vi "xijk_search_2D_table.vi"(8 "error in":errorcluster, 10 "sort array in":i32[](array[numeric]), 11 "all rows in":string[][](array[string])) -> (0 "error out":errorcluster, 3 "all rows out":string[][](array[string]))   [LabVIEW 2009, in "xijk_select_best_filter.lvlib"]
uses:
  xijk_select_best_filter.lvlib
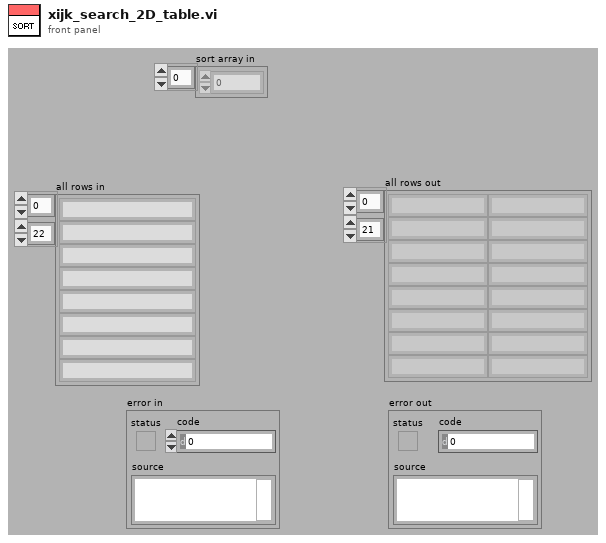
[diagram p1: front panel]
types:
  T1 = cluster{"all rows in[0]":string, "all rows in[1]":string, "all rows in[2]":string, "all rows in[3]":string, "all rows in[4]":string, "all rows in[5]":string, "all rows in[6]":string, "all rows in[7]":string, "all rows in[8]":string, "all rows in[9]":string, "all rows in[10]":string, "all rows in[11]":string, "all rows in[12]":string, "all rows in[13]":string, "all rows in[14]":string, "all rows in[15]":string, "all rows in[16]":string, "all rows in[17]":string, "all rows in[18]":string, "all rows in[19]":string, "all rows in[20]":string, "all rows in[21]":string, "all rows in[22]":string}
  T2 = cluster{"String":dbl, "all rows in":cluster{"all rows in[0]":string, "all rows in[1]":string, "all rows in[2]":string, "all rows in[3]":string, "all rows in[4]":string, "all rows in[5]":string, "all rows in[6]":string, "all rows in[7]":string, "all rows in[8]":string, "all rows in[9]":string, "all rows in[10]":string, "all rows in[11]":string, "all rows in[12]":string, "all rows in[13]":string, "all rows in[14]":string, "all rows in[15]":string, "all rows in[16]":string, "all rows in[17]":string, "all rows in[18]":string, "all rows in[19]":string, "all rows in[20]":string, "all rows in[21]":string, "all rows in[22]":string}}
  T3 = cluster{"String":dbl, "all rows in":cluster{"all rows in[0]":string, "all rows in[1]":string, "all rows in[2]":string, "all rows in[3]":string, "all rows in[4]":string, "all rows in[5]":string, "all rows in[6]":string, "all rows in[7]":string, "all rows in[8]":string, "all rows in[9]":string, "all rows in[10]":string, "all rows in[11]":string, "all rows in[12]":string, "all rows in[13]":string, "all rows in[14]":string, "all rows in[15]":string, "all rows in[16]":string, "all rows in[17]":string, "all rows in[18]":string, "all rows in[19]":string, "all rows in[20]":string, "all rows in[21]":string, "all rows in[22]":string}}[]
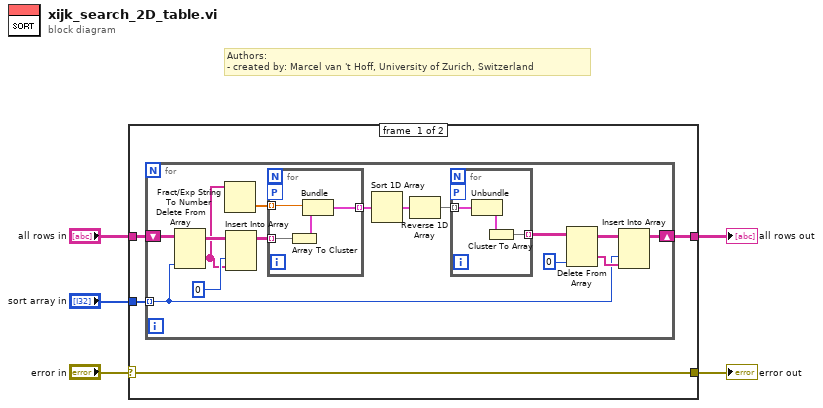
[diagram p0: block diagram]
diagram:
  # "Authors: \n- created by: Marcel van 't Hoff, University of Zurich, Switzerland"
  n1 = case shown="No Error" "error in" {
    selector: "error in" -> [w6 w32]
    tunnel: "sort array in" -> [w9 _]
    tunnel: "all rows in" -> [w8 _]
    tunnel: [w6 w32] -> w1
    tunnel: [w7 _] -> w2
    frame #0 {
      n2 = for {
        shift-right: [w16] -> w7
        shift-left: w8 -> [w13]
        tunnel: w9 -> [w14] mode=indexing
        n3 = Delete From Array(array=w13, index (col)=w14) -> (deleted portion=w12:string[], array with subset deleted=w22:string[][])  [unwired: 2 in]
        n4 = Fract/Exp String To Number(string=w12) -> (number=w11:dbl[])  [unwired: 3 in, 1 out]
        n5 = Insert Into Array(array=w22, index (col)=0 ("disabled index (col)"), new element=w12) -> (w17:string[][])  [unwired: 1 in]
        n6 = for {
          tunnel: w17 -> [w28] mode=indexing
          workers-P: _ -> [_]
          tunnel: w11 -> [w26] mode=indexing
          tunnel: [w25] -> w10 mode=indexing
          n7 = Array To Cluster(array=w28) -> (cluster=w27:T1)
          n8 = Bundle("String"=w26, "all rows in"=w27) -> (w25:T2)  [unwired: 1 in]
        }
        n9 = Sort 1D Array(array=w10) -> (sorted array=w23:T3)
        n10 = Reverse 1D Array(array=w23) -> (reversed array=w24:T3)
        n11 = for {
          tunnel: w24 -> [w30] mode=indexing
          tunnel: [w31] -> w15 mode=indexing
          workers-P: _ -> [_]
          n12 = Unbundle(w30) -> ("all rows in"=w29:T1)  [unwired: 1 out]
          n13 = Cluster To Array(cluster=w29) -> (array=w31:string[])
        }
        n14 = Delete From Array(array=w15, index (col)=0 ("disabled index (col)")) -> (deleted portion=w18:string[], array with subset deleted=w19:string[][])  [unwired: 2 in]
        n15 = Insert Into Array(array=w19, index (col)=w14, new element=w18) -> (w16:string[][])  [unwired: 1 in]
      }
    }
    frame #1 {
    }
  }
  "error out" <- w1
  "all rows out" <- w2
